vi "未命名 2.vi"() -> ()   [LabVIEW 2018]
uses:
  <vilib>/Utility/miscctls.llb/LVBoundsTypeDef.ctl
  <vilib>/picture/picture.llb/Draw 1-Bit Pixmap.vi
  <vilib>/Utility/NIReport.llb/Report Type.ctl
  <vilib>/Utility/NIReport.llb/image depth.ctl
  <vilib>/Utility/NIReport.llb/NI_ReportGenerationCore.lvlib
  <vilib>/Utility/NIReport.llb/NI_report.lvclass
panel:
  in  "Text":string="31S5106            W84B9L004        20180419SBDCNMR-JE-70B                      0001"
  in  "ErrorCorrectLevel":i32(ring) items=["L", "M", "Q", "H"]
  in  "Scale":u8=4
  out "绘图区域大小":T1
  out "new picture":picture caption="新图片"
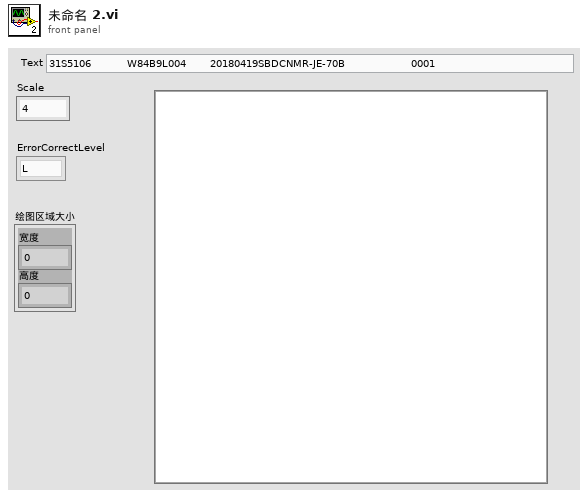
[diagram p1: front panel]
types:
  T1 = typedef "LVBoundsTypeDef.ctl" = cluster{"Width":u32, "Height":u32}
  T2 = typedef "NI_ReportGenerationCore.lvlib/Report Type.ctl" = enum16{"HTML", "Word", "Excel"}
  T3 = typedef "NI_ReportGenerationCore.lvlib/image depth.ctl" = u16
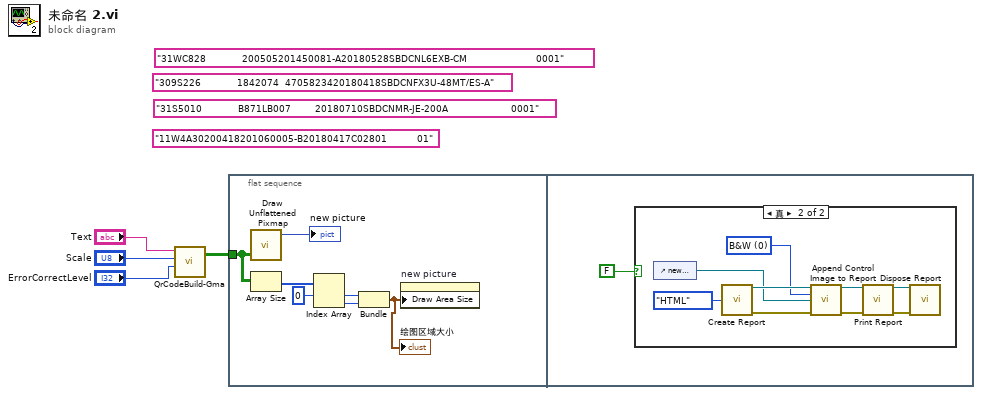
[diagram p0: block diagram]
diagram:
  (unwired) "11W4A30200418201060005-B20180417C02801          01"
  (unwired) "31S5010            B871LB007        20180710SBDCNMR-JE-200A                     0001"
  (unwired) "309S226            1842074  4705823420180418SBDCNFX3U-48MT/ES-A"
  (unwired) "31WC828            200505201450081-A20180528SBDCNL6EXB-CM                       0001" ("Text")
  n1 = call "QrCodeBuild-Gma.vi"("ErrorCorrectLevel"="ErrorCorrectLevel", "Scale(4)"="Scale", "Text"="Text") -> ("out Array"=w4:bool[][])  [unwired: 2 in]
  n2 = flat-sequence {
    tunnel: w4 -> [w10]
    frame #0 {
      n3 = call-poly <vilib>:"Draw Unflattened Pixmap.vi"("data"=w10) -> ("new picture"=→"new picture":picture)  [unwired: 8 in]
      n4 = Array Size(array=w10) -> (size(s)=w9:i32[])
      n5 = Index Array(array=w9, index #1=0 ("索引")) -> (element #1=w6:i32, element #2=w7:i32)  [unwired: 1 in]
      n6 = Bundle(w6, w7) -> (w5:cluster{i32, i32})  [unwired: 1 in]
      "绘图区域大小" <- w5
      n7 = property on="new picture" class="Pict"("Draw Area Size"=w5) -> ()  [unwired: 2 in, 2 out]
    }
    frame #1 {
      n8 = case shown="真" FALSE {
        frame False {
        }
        frame True {
          w14 = T3 0 items=["B&W", "4 bits", "8 bits", "24 bits"] ("image depth")
          n9 = control-ref of="new picture"() -> (w13:refnum<vi>)
          n10 = call <vilib>:"Create Report.vi"("report type"=Report_Type."HTML") -> ("report out"=w20:refnum<class "NI_report.lvclass">, "error out"=w19:errorcluster)  [unwired: 13 in]
          n11 = call-dynamic "Append Control Image to Report.vi"("report in"=w20, "image depth"=w14, "ctrl reference"=w13, "error in (no error)"=w19) -> ("report out"=w18:refnum<class "NI_report.lvclass">, "error out"=w17:errorcluster)  [unwired: 8 in, 2 out]
          n12 = call-dynamic "Print Report.vi"("report in"=w18, "error in (no error)"=w17) -> ("report out"=w16:refnum<class "NI_report.lvclass">, "error out"=w15:errorcluster)  [unwired: 12 in]
          n13 = call-dynamic "Dispose Report.vi"("report in"=w16, "error in (no error)"=w15) -> ()  [unwired: 13 in, 1 out]
        }
      }
    }
  }
